vi "Create Template Settings.vi"(8 "error in (no error)":errorcluster, 10 "Name":string, 11 "Acrobat Template in":refnum<class "Application.lvclass">) -> (0 "error out":errorcluster, 3 "Acrobat Template out":refnum<class "Application.lvclass">)   [LabVIEW 2015, in "Application.lvlib" / "Application.lvclass"]
uses:
  Application.lvclass
  Settings/App Settings.lvclass
  Application.lvclass/Application.ctl
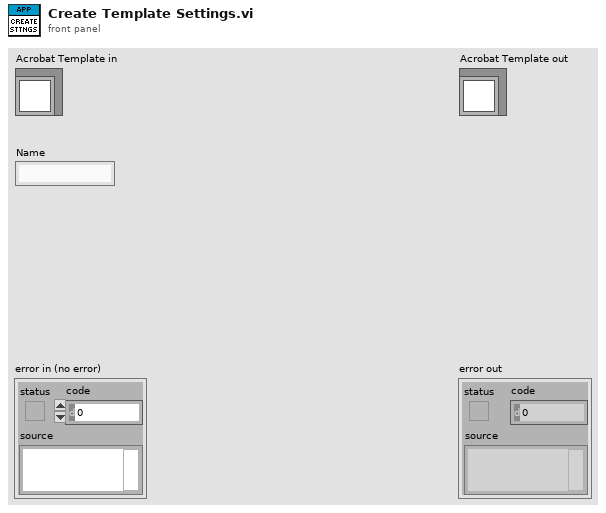
[diagram p1: front panel]
types:
  T1 = typedef "Application.lvlib/App Settings.lvclass/Class Settings -- Cluster.ctl" = cluster{"MES Enabled":bool, "DataLogging Enabled":bool, "AutoStart":bool, "AutoClear":bool, "Cycle Timeout":u32, "Wait Before Clear":u32, "Machine ID":string, "Test Type":string, "Product Name":string, "Meta Tags":string[], "Meta Values":string[], "Viewer Settings":cluster{"DataViewer Headers":string[], "Pass Fail Settings":T2}}
  T2 = typedef "Data Viewer.lvlib/Data Viewer Settings.lvclass/Pass Fail Criteria -- Cluster.ctl" = cluster{"Header":string, "Criteria":string}
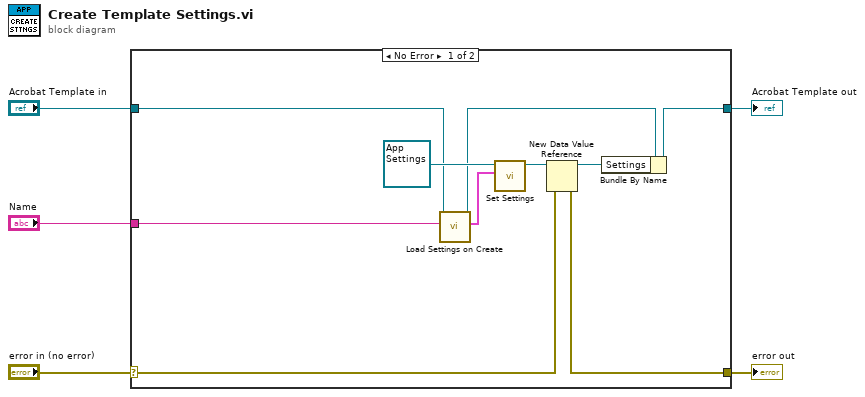
[diagram p0: block diagram]
diagram:
  n1 = case shown="No Error" "error in (no error)" {
    selector: "error in (no error)" -> [w14 w17]
    tunnel: [w13 w17] -> w4
    tunnel: [w15 w16] -> w2
    tunnel: "Acrobat Template in" -> [w9 w16]
    tunnel: "Name" -> [w7 _]
    frame No Error {
      n2 = call "Load Settings on Create.vi"("Name"=w7, "Application in"=w9) -> ("Settings"=w6:T1, "Application out"=w8:refnum<class "Application.lvclass">)  [unwired: 7 in, 1 out]
      n3 = call-dynamic "Set Settings.vi"("Settings"=w6, "App Settings in"=refnum<class "App Settings.lvclass"> refnum ("Application.lvlib:App Settings.lvclass")) -> ("App Settings out"=w10:refnum<class "App Settings.lvclass">)  [unwired: 8 in, 1 out]
      n4 = New Data Value Reference(data value=w10, error in=w14) -> (data value reference=w12:refnum<data-value>, error out=w13:errorcluster)
      n5 = Bundle By Name(cluster=w8, "Settings"=w12) -> (w15:refnum<class "Application.lvclass">)
    }
    frame Error {
    }
  }
  "error out" <- w4
  "Acrobat Template out" <- w2
